vi "Enable Item.vi"(8 "error in (no error)":errorcluster caption="错误输入（无错误）", 9 "Item Name":string, 10 "Module Name":string, 11 "User Interface 输入":refnum<class "User Interface.lvclass">) -> (0 "error out":errorcluster caption="错误输出", 3 "User Interface 输出":refnum<class "User Interface.lvclass">)   [LabVIEW 2018, in "MainInterface.lvlib" / "User Interface.lvclass"]
uses:
  User Interface.lvclass
  User Interface.lvclass/User Interface.ctl
  ModuleInterface/ModuleInterface.lvlib
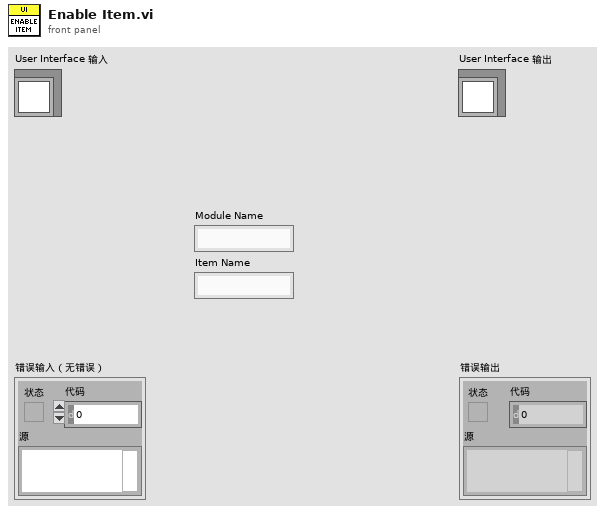
[diagram p1: front panel]
types:
  T1 = typedef "MainInterface.lvlib/User Interface.lvclass/Module Information.ctl" = cluster{"Module ID":i32, "Module Name":string}
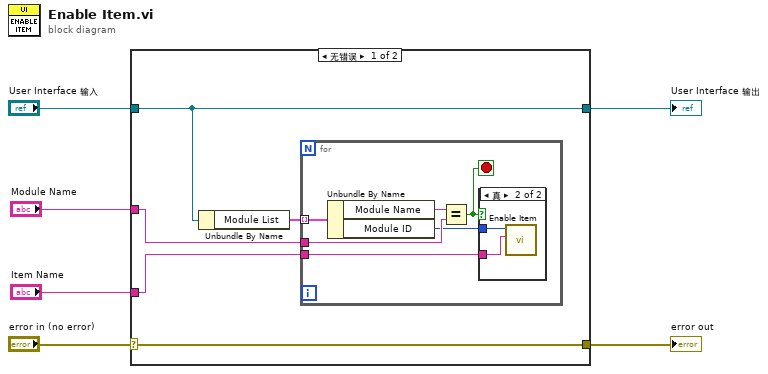
[diagram p0: block diagram]
diagram:
  n1 = case shown="无错误" "error in (no error)" {
    selector: "error in (no error)" -> [w11 w21]
    tunnel: [w11 w21] -> w5
    tunnel: [w10 w20] -> w3
    tunnel: "User Interface 输入" -> [w10 w20]
    tunnel: "Module Name" -> [w8 _]
    tunnel: "Item Name" -> [w7 _]
    frame No Error {
      n2 = Unbundle By Name(w10) -> ("Module List"=w9:T1[])
      n3 = for {
        tunnel: w9 -> [w17] mode=indexing
        tunnel: w8 -> [w15]
        tunnel: w7 -> [w12]
        stop <- w14 stop-if-true
        n4 = Unbundle By Name(w17) -> ("Module Name"=w16:string, "Module ID"=w13:i32)
        n5 = Equal?(x=w16, y=w15) -> (x = y?=w14:bool)
        n6 = case shown="真" w14 {
          tunnel: w13 -> [_ w18]
          tunnel: w12 -> [_ w19]
          frame False {
          }
          frame True {
            n7 = call "Enable Item.vi"("Item Name"=w19, "Module ID"=w18) -> ()  [unwired: 9 in, 1 out]
          }
        }
      }
    }
    frame Error {
    }
  }
  "error out" <- w5
  "User Interface 输出" <- w3
